vi "Delayed Send to Consumer.vi"(7 "Seconds (5)":dbl=5.0, 8 "error in (no error)":errorcluster, 9 "Data":variant, 10 "Case ID":variant, 11 "Father of all uServices in":refnum<class "Father of all uServices.lvclass">) -> (0 "error out":errorcluster, 3 "Father of all uServices out":refnum<class "Father of all uServices.lvclass">)   [LabVIEW 2026, in "TALOS.lvlib" / "Father of all uServices.lvlib" / "Father of all uServices.lvclass"]
doc: "VI for sending delayed message to the Consumer"
uses:
  Father of all uServices.lvclass
  C:/LabVIEW Code/TALOS/builds/Actor Framework PPL/Actor Framework.lvlibp/1abvi3w/vi.lib/ActorFramework/Actor/Actor.lvclass
  Father of all uServices Messages/Consumer Msg/Consumer Msg.lvclass/Consumer Msg.ctl
  Ancestor/Ancestor/Ancestor.lvclass/Ancestor.ctl
  Father of all uServices Messages/Consumer Msg/Send Consumer.vi
  Support VIs/Generate Error.vi
  FGV/Error Memory/Get Error Description.vi
  Support VIs/Get PC name.vi
  Ancestor/Ancestor/Read ID.vi
  Support VIs/Get Class Name.vi
  <vilib>/Utility/error.llb/Clear Errors.vi
  FGV/Error Memory/Error Memory Core.vi
  <vilib>/AdvancedString/Delimited String to 1D String Array.vi
  <vilib>/AdvancedString/Delimited String to 1D String Array (string).vi
  Support VIs/Circus Root Path.vi
  FGV/Error Memory/Error Crt Lvl checker.vi
  FGV/Error Memory/Error Memory Core.vi/40c8088d-b597-4017-91af-faa98e00292e.vi
  FGV/Error Memory/Error Memory Core.vi/d4a3ab98-063c-4e44-b43d-fbdcfe6c2be2.vi
  builds/Actor Framework PPL/Actor Framework.lvlibp/1abvi3w/vi.lib/ActorFramework/Actor/Read Self Enqueuer.vi
  <userlib>/_OpenG.lib/lvdata/lvdata.llb/Get Strings from Enum__ogtk.vi
  builds/Actor Framework PPL/Actor Framework.lvlibp/1abvi3w/vi.lib/ActorFramework/Message Enqueuer/Enqueue.vi
  Support VIs/Global Memory.vi
  <vilib>/Utility/LVClass/Get LV Class Name.vi
  Support VIs/Is in Packed Library.vi
  Support VIs/TALOS Root path.vi
  Support VIs/Read CSV worksheet.vi
  Support VIs/Global Constants.vi
  <vilib>/Utility/error.llb/General Error Handler.vi
  Support VIs/Error Log.vi
  Delayed Send to Consumer - Core.vi
  Father of all uServices Messages/Consumer Msg/Consumer Msg.lvclass
  Ancestor/Ancestor/Ancestor.lvclass
  <vilib>/Comparison/Equal/Equal Functor/Equal Functor.lvclass
  TALOS.lvlib
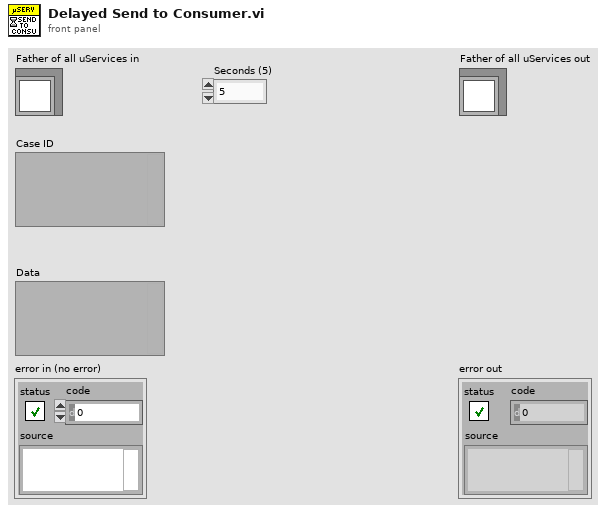
[diagram p1: front panel]
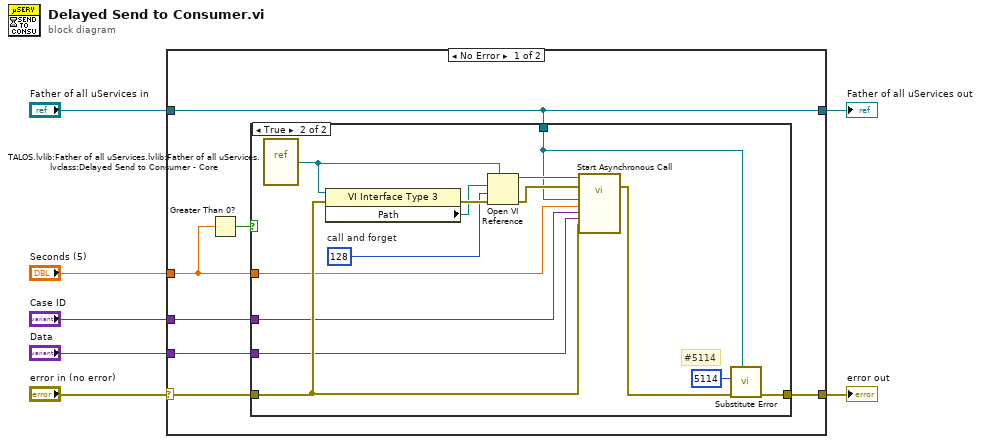
[diagram p0: block diagram]
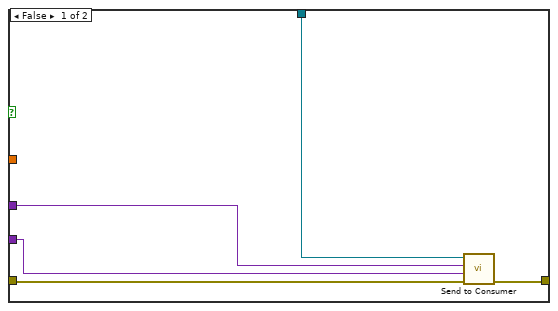
[diagram p2: hidden frame]
diagram:
  n1 = case shown="No Error" "error in (no error)" {
    selector: "error in (no error)" -> [w14 w35]
    tunnel: [w11 w35] -> w6
    tunnel: [w10 w34] -> w4
    tunnel: "Father of all uServices in" -> [w10 w34]
    tunnel: "Case ID" -> [w12 _]
    tunnel: "Data" -> [w13 _]
    tunnel: "Seconds (5)" -> [w9 _]
    frame No Error {
      n2 = Greater Than 0?(x=w9) -> (x > 0?=w8:bool)
      n3 = case shown="True" w8 {
        tunnel: w14 -> [w18 w33]
        tunnel: w9 -> [_ w27]
        tunnel: w13 -> [w15 w26]
        tunnel: w12 -> [w16 w25]
        tunnel: [w19 w23] -> w11
        tunnel: w10 -> [w17 w21]
        frame False {
          n4 = call "Send to Consumer.vi"("error in (no error)"=w18, "Data"=w15, "Case ID"=w16, "uService Template in"=w17) -> ("error out"=w19:errorcluster)  [unwired: 6 in, 1 out]
        }
        frame True {
          w31 = 128  # call and forget
          # "#5114"
          n5 = vi-ref "TALOS.lvlib:Father of all uServices.lvlib:Father of all uServices.lvclass:Delayed Send to Consumer - Core.vi"() -> (w20:refnum<vi>)
          n6 = property class="VI Interface Type 3"(reference=w20, error in=w33) -> (error out=w32:errorcluster, "Path"=w30:path)  [unwired: 1 out]
          n7 = Open VI Reference(type specifier VI Refnum (for type only)=w20, vi path=w30, options=w31, error in (no error)=w32) -> (vi reference=w28:refnum<vi>, error out=w29:errorcluster)  [unwired: 2 in]
          n8 = call-by-ref "Start Asynchronous Call"(reference=w28, error in=w29, "Father of all uServices in"=w21, "Seconds"=w27, "Case ID"=w25, "Data"=w26, 11:"error in (no error)"=w33) -> (error out=w24:errorcluster)  [unwired: 9 in, 3 out]
          n9 = call "Substitute Error.vi"("LabVIEW Object"=w21, "error in (no error)"=w24, "Error Code"=5114) -> ("error out"=w23:errorcluster)  [unwired: 8 in]
        }
      }
    }
    frame Error {
    }
  }
  "error out" <- w6
  "Father of all uServices out" <- w4
